vi "ReadSystemDefinitionOverrideFile.vi"(8 "error in (no error)":errorcluster, 11 "configuration file path":path) -> (0 "error out":errorcluster, 3 "modifier items":T1[](array[typedef]))   [LabVIEW 2015, in "VeriStandTestUtilities.lvlib"]
uses:
  VeriStandTestUtilities.lvlib
  ConfigurationItem.ctl
  ConfigurationItemType.ctl
  OverrideItem.ctl
  <vilib>/Utility/config.llb/Read Key (String).vi
  <vilib>/Utility/config.llb/NI_LVConfig.lvlib
panel:
  in  "modifier item":T1
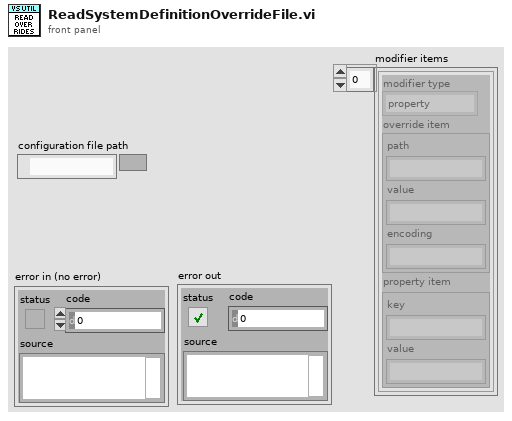
[diagram p1: front panel]
types:
  T1 = typedef "VeriStandTestUtilities.lvlib/ConfigurationItem.ctl" = cluster{"modifier type":T2, "override item":T3, "property item":cluster{"key":string, "value":string}}
  T2 = typedef "VeriStandTestUtilities.lvlib/ConfigurationItemType.ctl" = enum16{"property", "override"}
  T3 = typedef "VeriStandTestUtilities.lvlib/OverrideItem.ctl" = cluster{"path":string, "value":string, "encoding":string}
  T4 = typedef "NI_LVConfig.lvlib/Config Data RefNum.ctl" = refnum<k1>
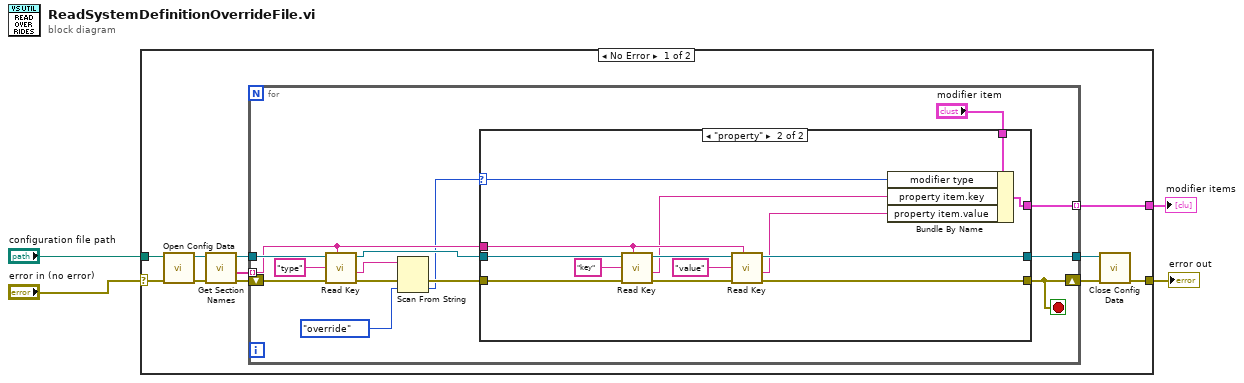
[diagram p0: block diagram]
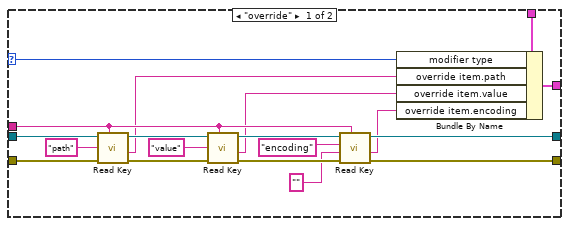
[diagram p2: hidden frame]
diagram:
  n1 = case shown="No Error" "error in (no error)" {
    selector: "error in (no error)" -> [w6 w63]
    tunnel: [w15 w63] -> w4
    tunnel: "configuration file path" -> [w14 _]
    tunnel: [w5 _] -> w1
    frame No Error {
      n2 = call <vilib>:"Open Config Data.vi"("error in (no error)"=w6, "configuration file path"=w14) -> ("error out"=w7:errorcluster, "refnum"=w8:T4)  [unwired: 7 in, 1 out]
      n3 = call <vilib>:"Get Section Names.vi"("error in (no error)"=w7, "refnum"=w8) -> ("error out"=w11:errorcluster, "section names"=w9:string[], "refnum out"=w10:T4)  [unwired: 7 in]
      n4 = for {
        tunnel: w9 -> [w22] mode=indexing
        tunnel: w10 -> [w24]
        tunnel: [w27] -> w12
        tunnel: [w28] -> w5 mode=indexing
        shift-right: [w29] -> w13
        shift-left: w11 -> [w25]
        stop <- w29 stop-if-true
        n5 = call-poly <vilib>:"Read Key.vi"("section"=w22, "error in (no error)"=w25, "key"="type", "refnum"=w24) -> ("error out"=w21:errorcluster, "value"=w18:string, "refnum out"=w23:T4)  [unwired: 4 in, 1 out]
        n6 = Scan From String(input string=w18, error in=w21, default 1=ConfigurationItemType."override" ("modifier type")) -> (error out=w20:errorcluster, output 1=w17:T2)  [unwired: 2 in, 2 out]
        n7 = case shown="\"property\"" w17 {
          selector: w17 -> [w30 w60]
          tunnel: [w43 w52] -> w29
          tunnel: [w34 w61] -> w28
          tunnel: [w39 w53] -> w27
          tunnel: w20 -> [w38 w55]
          tunnel: w23 -> [w37 w54]
          tunnel: w22 -> [w36 w51]
          tunnel: "modifier item" -> [w35 w62]
          frame "override" {
            n8 = call-poly <vilib>:"Read Key.vi"("section"=w36, "error in (no error)"=w38, "key"="path", "refnum"=w37) -> ("error out"=w47:errorcluster, "value"=w31:string, "refnum out"=w46:T4)  [unwired: 4 in, 1 out]
            n9 = call-poly <vilib>:"Read Key.vi"("section"=w36, "error in (no error)"=w47, "key"="value", "refnum"=w46) -> ("error out"=w44:errorcluster, "value"=w32:string, "refnum out"=w40:T4)  [unwired: 4 in, 1 out]
            n10 = call-poly <vilib>:"Read Key.vi"("section"=w36, "error in (no error)"=w44, "default value"="", "key"="encoding", "refnum"=w40) -> ("error out"=w43:errorcluster, "value"=w33:string, "refnum out"=w39:T4)  [unwired: 3 in, 1 out]
            n11 = Bundle By Name(cluster=w35, "modifier type"=w30, "override item.path"=w31, "override item.value"=w32, "override item.encoding"=w33) -> (w34:T1)
          }
          frame "property" {
            n12 = call-poly <vilib>:"Read Key.vi"("section"=w51, "error in (no error)"=w55, "key"="key", "refnum"=w54) -> ("error out"=w58:errorcluster, "value"=w50:string, "refnum out"=w57:T4)  [unwired: 4 in, 1 out]
            n13 = call-poly <vilib>:"Read Key.vi"("section"=w51, "error in (no error)"=w58, "key"="value", "refnum"=w57) -> ("error out"=w52:errorcluster, "value"=w49:string, "refnum out"=w53:T4)  [unwired: 4 in, 1 out]
            n14 = Bundle By Name(cluster=w62, "modifier type"=w60, "property item.key"=w50, "property item.value"=w49) -> (w61:T1)
          }
        }
      }
      n15 = call <vilib>:"Close Config Data.vi"("error in (no error)"=w13, "refnum"=w12) -> ("error out"=w15:errorcluster)  [unwired: 8 in, 1 out]
    }
    frame Error {
    }
  }
  "error out" <- w4
  "modifier items" <- w1
